vi "Analyse input string for terminal.vi"(3 "Last string sent":string, 4 "String new":string) -> (14 "String out":string, 15 "Out not equal to in?":bool, 16 "Attach term. char.?":bool)   [LabVIEW 2026]
doc: "This VI is a sub-VI for PI Terminal.vi. It analyses String new and returns it in String out if it is not empty and does not contain a \"#\" at the beginning. In case of an empty new string, Last string sent is returned. If String new contains a \"#\" character, the corresponding ASCII character is returned."
panel:
  # "This vi is a sub-vi for\" PI Terminal.vi\". It analyses \"String new\" and returns it in \"String out\" if it is not empty and does not contain a \"#\" at the beginning. In case of an empty new string, \"Last string sent\" is returned. If \"String new\" contains a \"#\" character, the corresponding ASCII character is returned."
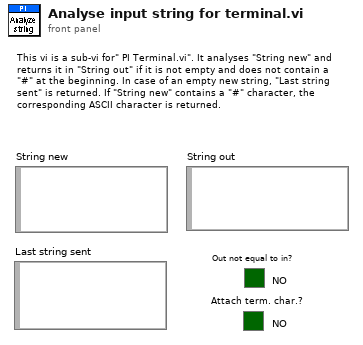
[diagram p1: front panel]
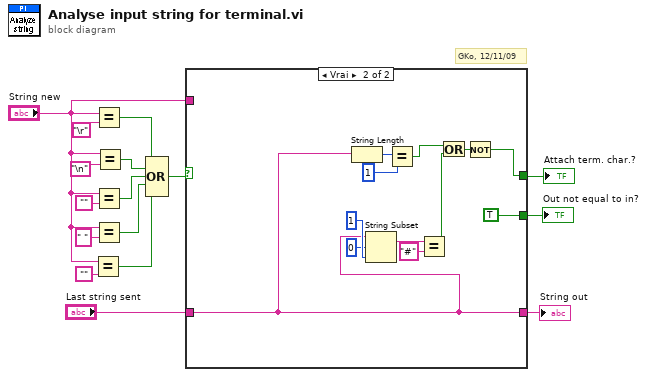
[diagram p0: block diagram]
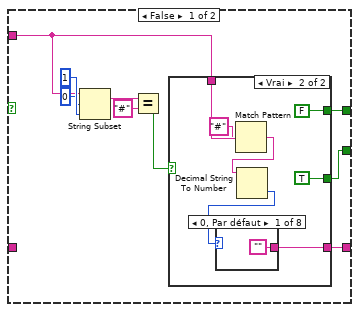
[diagram p2: hidden frame]
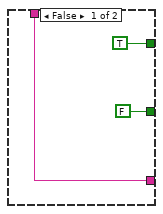
[diagram p3: hidden frame]
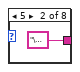
[diagram p4: hidden frame]
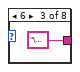
[diagram p5: hidden frame]
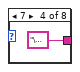
[diagram p6: hidden frame]
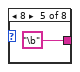
[diagram p7: hidden frame]
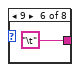
[diagram p8: hidden frame]
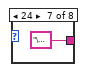
[diagram p9: hidden frame]
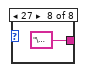
[diagram p10: hidden frame]
diagram:
  # "GKo, 12/11/09"
  n1 = Equal?(x="String new", y="") -> (x = y?=w6:bool)
  n2 = Equal?(x="String new", y="\r") -> (x = y?=w12:bool)
  n3 = Equal?(x="String new", y="") -> (x = y?=w10:bool)
  n4 = Equal?(x="String new", y=" ") -> (x = y?=w7:bool)
  n5 = Equal?(x="String new", y="\n") -> (x = y?=w11:bool)
  n6 = Compound Arithmetic op=OR(w12, w11, w10, w7, w6) -> (w9:bool)
  n7 = case shown="Vrai" w9 {
    tunnel: "String new" -> [w20 _]
    tunnel: [w19 TRUE ("Out not equal to in?")] -> w4
    tunnel: [w18 w49] -> w3
    tunnel: [w17 w44] -> w2
    tunnel: "Last string sent" -> [_ w49]
    frame False {
      n8 = String Subset(string=w20, offset (0)=0, length (rest)=1 ("length")) -> (substring=w23:string)
      n9 = Equal?(x=w23, y="#") -> (x = y?=w21:bool)
      n10 = case shown="Vrai" w21 {
        tunnel: w20 -> [w27 w35]
        tunnel: [FALSE TRUE] -> w19
        tunnel: [w27 w30] -> w18
        tunnel: [TRUE FALSE] -> w17
        frame False {
        }
        frame True {
          n11 = Match Pattern(string=w35, regular expression="#") -> (after substring=w32:string)  [unwired: 4 out]
          n12 = Decimal String To Number(string=w32) -> (number=w31:i32)  [unwired: 3 out]
          n13 = case shown="0, Par défaut" w31 {
            tunnel: ["" "\u0005" "\u0006" "\u0007" "\b" "\t" "\u0018" "\u001b"] -> w30
            frame 0, Default {
            }
            frame 5 {
            }
            frame 6 {
            }
            frame 7 {
            }
            frame 8 {
            }
            frame 9 {
            }
            frame 24 {
            }
            frame 27 {
            }
          }
        }
      }
    }
    frame True {
      n14 = String Length(string=w49) -> (length=w48:i32)
      n15 = String Subset(string=w49, offset (0)=0, length (rest)=1 ("length")) -> (substring=w52:string)
      n16 = Equal?(x=w48, y=1) -> (x = y?=w46:bool)
      n17 = Equal?(x=w52, y="#") -> (x = y?=w45:bool)
      n18 = Or(x=w46, y=w45) -> (x .or. y?=w50:bool)
      n19 = Not(x=w50) -> (.not. x?=w44:bool)
    }
  }
  "String out" <- w3
  "Out not equal to in?" <- w4
  "Attach term. char.?" <- w2
